vi "Prix_MP.vi"() -> ()   [LabVIEW 2024]
panel:
  in  "Prix_MP":dbl
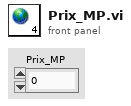
[diagram p1: front panel]
diagram:
